vi "Fail.vi"(8 "error in (no error)":errorcluster, 9 "Message (\"\")":string, 10 "Actual":variant, 11 "Constraint in":refnum<class "Constraint.lvclass">) -> (0 "error out":errorcluster, 3 "Constraint out":refnum<class "Constraint.lvclass">)   [LabVIEW 2017, in "Constraint.lvlib" / "Constraint.lvclass"]
doc: "Generates an error for the given value. Optionally adds a message."
uses:
  Constraint.lvclass
  Framework/LVUnit Test Framework/LVUnit Test Framework.lvclass
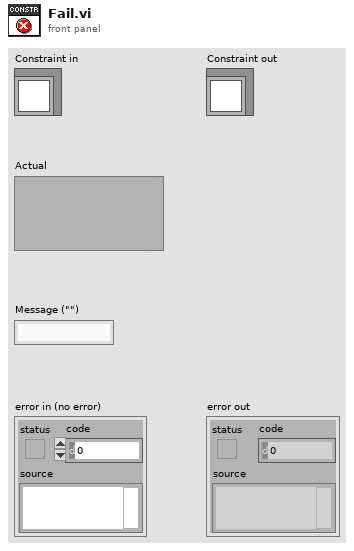
[diagram p1: front panel]
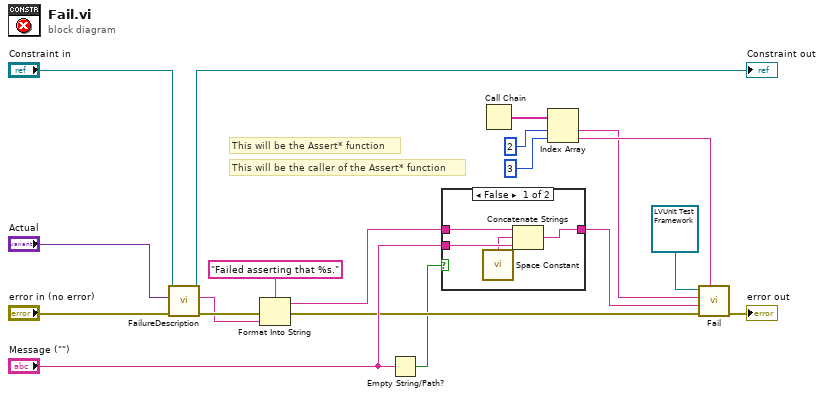
[diagram p0: block diagram]
diagram:
  # "This will be the Assert* function"
  # "This will be the caller of the Assert* function"
  n1 = call-dynamic "FailureDescription.vi"("error in (no error)"="error in (no error)", "Actual"="Actual", "Constraint in"="Constraint in") -> ("error out"=w11:errorcluster, "Failure Description"=w10:string, "Constraint out"=→"Constraint out":refnum<class "Constraint.lvclass">)  [unwired: 6 in]
  n2 = Format Into String(format string="Failed asserting that %s.", error in=w11, w10) -> (resulting string=w9:string, error out=w12:errorcluster)  [unwired: 1 in]
  n3 = Empty String/Path?(string/path="Message (\"\")") -> (empty?=w8:bool)
  n4 = case shown="False" w8 {
    tunnel: "Message (\"\")" -> [w23 _]
    tunnel: w9 -> [w21 w24]
    tunnel: [w20 w24] -> w7
    frame False {
      n5 = call <vilib>:"Space Constant.vi"() -> ("String"=w22:string)
      n6 = Concatenate Strings(w21, w22, w23) -> (w20:string)
    }
    frame True {
    }
  }
  n7 = Call Chain() -> (call chain=w6:string[])
  n8 = Index Array(array=w6, index #1=2 ("index"), index #2=3 ("index")) -> (element #1=w1:string, element #2=w5:string)
  n9 = call-dynamic "Fail.vi"("Caller"=w5, "error in (no error)"=w12, "Message"=w7, "Assertion"=w1, "LVUnit Test Framework in"=refnum<class "LVUnit Test Framework.lvclass"> refnum ("Framework.lvlib:LVUnit Test Framework.lvclass")) -> ("error out"=→"error out":errorcluster)  [unwired: 5 in, 1 out]
